vi "Display Error.vi"(8 "error in (no error)":errorcluster, 9 "LabActor Error":T1, 10 "Error message":string, 11 "Monitor-Pulse in":refnum<class "Application Controller.lvclass">) -> (0 "error out":errorcluster, 3 "Monitor-Pulse out":refnum<class "Application Controller.lvclass">)   [LabVIEW 2018, in "Application Controller.lvclass"]
uses:
  Application Controller.lvclass
  Template Module/LabActor Error.ctl
  <vilib>/Utility/error.llb/DialogType.ctl
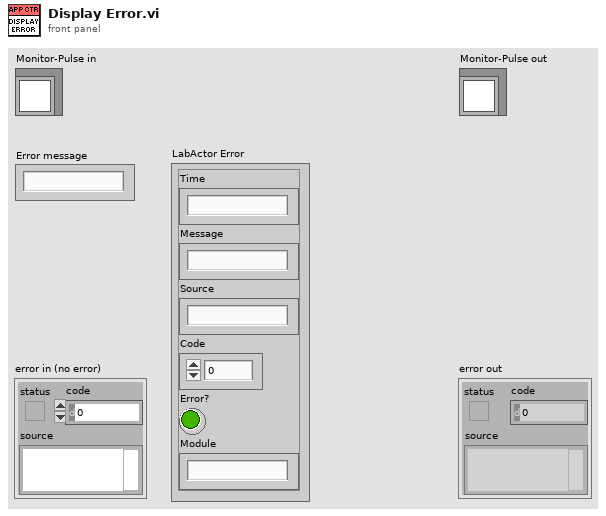
[diagram p1: front panel]
types:
  T1 = typedef "LabActor Error.ctl" = cluster{"Time":string, "Message":string, "Source":string, "Code":i32, "Error?":bool, "Module":string}
  T2 = typedef "DialogType.ctl" = u16
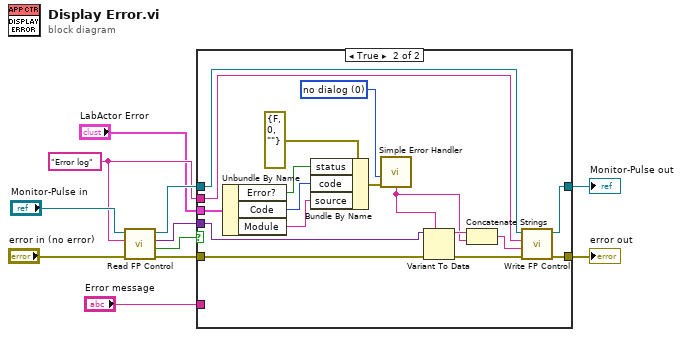
[diagram p0: block diagram]
diagram:
  w6 = "Error log" ("Control Name")
  n1 = call-dynamic "Read FP Control.vi"("error in (no error)"="error in (no error)", "Control Name"=w6, "Measure Object in"="Monitor-Pulse in") -> ("error out"=w9:errorcluster, "Present"=w2:bool, "Control Value"=w10:variant, "Measure Object out"=w7:refnum<class "Application Controller.lvclass">)  [unwired: 5 in]
  n2 = case shown="True" w2 {
    tunnel: w10 -> [_ w30]
    tunnel: w9 -> [w13 w29]
    tunnel: "Error message" -> [_ _]
    tunnel: w7 -> [w12 w27]
    tunnel: w6 -> [_ w26]
    tunnel: [w13 w23] -> w5
    tunnel: [w12 w22] -> w4
    tunnel: "LabActor Error" -> [_ w21]
    frame False {
    }
    frame True {
      w19 = T2 0 items=["no dialog", "OK message", "continue or stop message", "OK message + warnings", "continue/stop + warnings"] ("type of dialog (OK msg:1)")
      n3 = Unbundle By Name(w21) -> ("Error?"=w17:bool, "Code"=w16:i32, "Module"=w15:string)
      n4 = Bundle By Name(cluster=errorcluster {"status"=FALSE, "code"=0, "source"=""} ("error in (no error)"), "status"=w17, "code"=w16, "source"=w15) -> (w18:errorcluster)
      n5 = call <vilib>:"Simple Error Handler.vi"("type of dialog (OK msg:1)"=w19, "error in (no error)"=w18) -> ("message"=w14:string)  [unwired: 3 in, 4 out]
      n6 = Variant To Data(error in=w29, type=w14, Variant=w30) -> (data=w28:string, error out=w24:errorcluster)
      n7 = Concatenate Strings(w28, w14) -> (w25:string)
      n8 = call-dynamic "Write FP Control.vi"("error in (no error)"=w24, "Control Value"=w25, "Control Name"=w26, "Measure Object in"=w27) -> ("error out"=w23:errorcluster, "Measure Object out"=w22:refnum<class "Application Controller.lvclass">)  [unwired: 6 in]
    }
  }
  "error out" <- w5
  "Monitor-Pulse out" <- w4
